vi "Linear step array.vi"(8 "Step":dbl, 9 "End":dbl, 10 "Start":dbl, 11 "Mode":enum16{"Up", "Up-down"}(ring)) -> (3 "Steps":dbl[](array[numeric]))   [LabVIEW 2015]
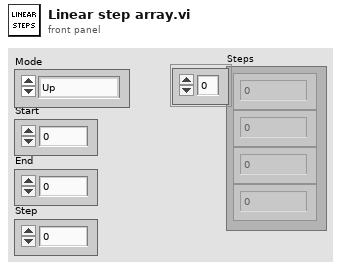
[diagram p1: front panel]
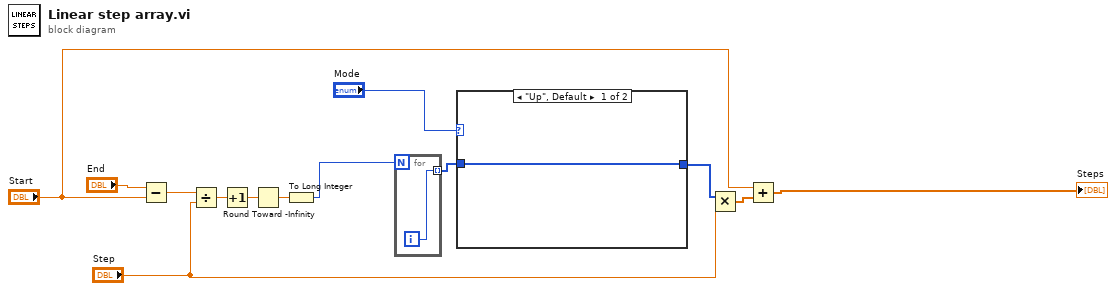
[diagram p0: block diagram]
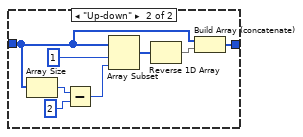
[diagram p2: hidden frame]
diagram:
  n1 = Subtract(x="End", y="Start") -> (x-y=w13:dbl)
  n2 = Divide(x=w13, y="Step") -> (x/y=w12:dbl)
  n3 = Increment(x=w12) -> (x+1=w11:dbl)
  n4 = Round Toward -Infinity(1:w11) -> (0:w10:dbl)
  n5 = To Long Integer(number=w10) -> (32bit integer=w8:i32)
  n6 = for {
    N: w8 -> [_]
    tunnel: [w14] -> w2 mode=indexing
    i -> [w14]
  }
  n7 = case shown="\"Up\", Default" "Mode" {
    tunnel: w2 -> [w15 w18]
    tunnel: [w15 w16] -> w1
    frame "Up", Default {
    }
    frame "Up-down" {
      n8 = Array Size(array=w18) -> (size(s)=w22:i32)
      n9 = Subtract(x=w22, y=2) -> (x-y=w20:i32)
      n10 = Array Subset(array=w18, index=1, length=w20) -> (w19:i32[])
      n11 = Reverse 1D Array(array=w19) -> (reversed array=w17:i32[])
      n12 = Build Array (concatenate)(w18, w17) -> (w16:i32[])
    }
  }
  n13 = Multiply(x=w1, y="Step") -> (x*y=w6:dbl[])
  n14 = Add(x="Start", y=w6) -> (x+y=→"Steps":dbl[])
